vi "web test string v1.vi"(10 "String2":string, 11 "String1":string) -> ()   [LabVIEW 2013]
panel:
  in  "Tab Control":enum32{"Page 1", "Page 2"}(tab)
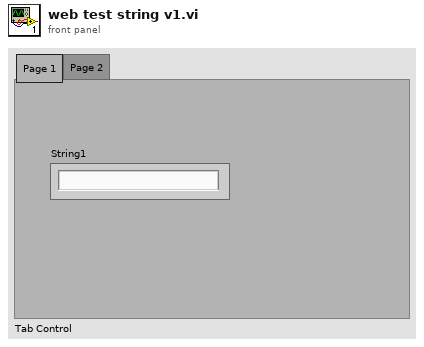
[diagram p1: front panel]
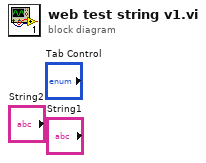
[diagram p0: block diagram]
diagram:
